vi "Parse Response (String).vi"(8 "error in":errorcluster, 10 "Response String In":string) -> (0 "error out":errorcluster, 1 "LabVIEW Error?":bool=TRUE, 2 "value":string)   [LabVIEW 2015, in "JSONRPC Server.lvclass"]
uses:
  JSONRPC Server.lvclass
  <vilib>/National Instruments/JSON Support for LabVIEW/JSON Data Classes/JSON Helper/To More Specific Type (String).vi
  <vilib>/National Instruments/JSON Support for LabVIEW/JSON Data Classes/JSON String/Read value (String).vi
  <vilib>/National Instruments/JSON Support for LabVIEW/JSON Data Classes/JSON Helper/JSON Helper.lvclass
  <vilib>/National Instruments/JSON Support for LabVIEW/JSON Data Classes/JSON Basic Type/JSON Literal.lvclass
  <vilib>/National Instruments/JSON Support for LabVIEW/JSON Data Classes/JSON String/JSON String.lvclass
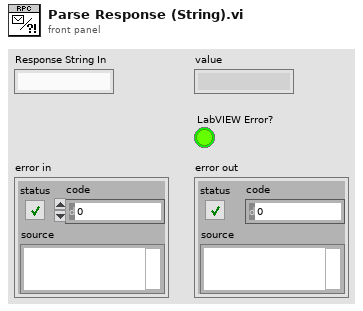
[diagram p1: front panel]
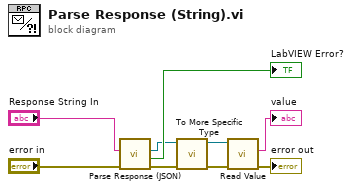
[diagram p0: block diagram]
diagram:
  n1 = call "Parse Response (JSON).vi"("error in"="error in", "Response String In"="Response String In") -> ("error out"=w5:errorcluster, "LabVIEW Error?"=→"LabVIEW Error?":bool, "JSON out"=w6:refnum<class "JSON Null.lvclass">)  [unwired: 7 in]
  n2 = call-poly <vilib>:"To More Specific Type.vi"("error in (no error)"=w5, "JSON Datatype in"=w6) -> ("error out"=w1:errorcluster, "JSON Datatype out"=w4:refnum<class "JSON String.lvclass">)  [unwired: 8 in]
  n3 = call-poly <vilib>:"Read Value.vi"("error in (no error)"=w1, "JSON String in"=w4) -> ("error out"=→"error out":errorcluster, "value"=→"value":string)  [unwired: 8 in]
